vi "GenerateLeftRight.vi"(10 "TrackWidth":dbl=20.0, 11 "SmoothPath":dbl[][](array[numeric])) -> (1 "Right":dbl[][](array[numeric]), 2 "Left":dbl[][](array[numeric]), 3 "Heading":dbl[](array[numeric]))   [LabVIEW 2016]
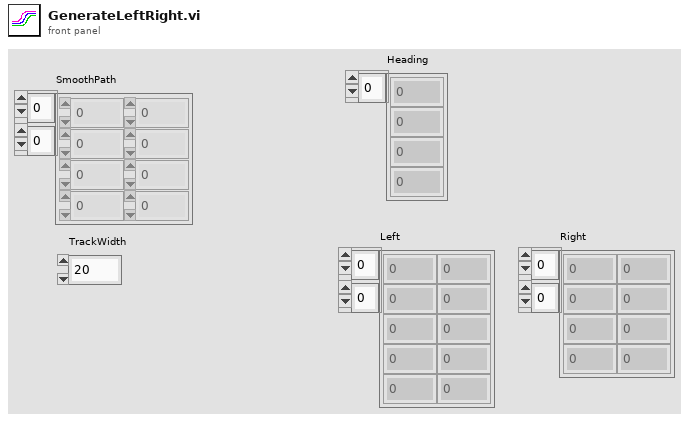
[diagram p1: front panel]
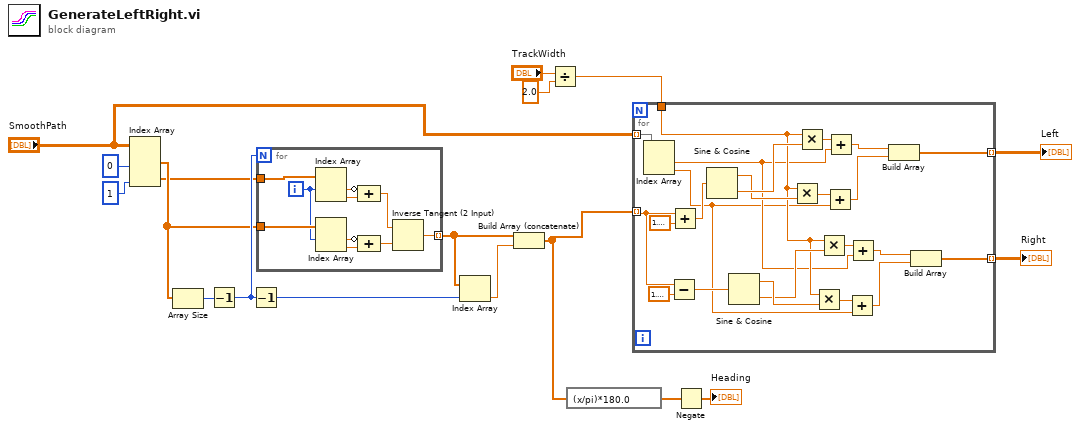
[diagram p0: block diagram]
diagram:
  n1 = Index Array(array="SmoothPath", index (col) #1=0 ("disabled index (col)"), index (col) #2=1 ("index (col)")) -> (element #1=w13:dbl[], element #2=w12:dbl[])  [unwired: 2 in]
  n2 = Array Size(array=w13) -> (size(s)=w17:i32)
  n3 = Decrement(x=w17) -> (x-1=w15:i32)
  n4 = Decrement(x=w15) -> (x-1=w14:i32)
  n5 = for {
    N: w15 -> [_]
    tunnel: w13 -> [w28]
    tunnel: w12 -> [w27]
    tunnel: [w20] -> w5 mode=indexing
    i -> [w19]
    n6 = Index Array(array=w27, index #1=w19) -> (element #1=w25:dbl, element #2=w26:dbl)  [unwired: 1 in]
    n7 = Index Array(array=w28, index #1=w19) -> (element #1=w23:dbl, element #2=w24:dbl)  [unwired: 1 in]
    n8 = Compound Arithmetic op=ADD(invert w25, w26) -> (w22:dbl)
    n9 = Compound Arithmetic op=ADD(invert w23, w24) -> (w21:dbl)
    n10 = Inverse Tangent (2 Input)(1:w21, 2:w22) -> (0:w20:dbl)
  }
  n11 = Index Array(array=w5, index=w14) -> (element=w4:dbl)
  n12 = Build Array (concatenate)(w5, w4) -> (w3:dbl[])
  n13 = Divide(x="TrackWidth", y=2.0) -> (x/y=w9:dbl)
  n14 = expression code="(x/pi)*180.0" ("radians to degrees")(w3) -> (w2:dbl[])
  n15 = for {
    tunnel: w3 -> [w33] mode=indexing
    tunnel: w9 -> [w32]
    tunnel: "SmoothPath" -> [w34] mode=indexing
    tunnel: [w43] -> w7 mode=indexing
    tunnel: [w31] -> w6 mode=indexing
    n16 = Index Array(array=w34) -> (element #1=w30:dbl, element #2=w29:dbl)  [unwired: 2 in]
    n17 = Subtract(x=w33, y=1.5707963267948966) -> (x-y=w36:dbl)
    n18 = Add(x=w33, y=1.5707963267948966) -> (x+y=w50:dbl)
    n19 = Sine & Cosine(0:w50) -> (1:w46:dbl, 2:w47:dbl)
    n20 = Sine & Cosine(0:w36) -> (1:w40:dbl, 2:w39:dbl)
    n21 = Multiply(x=w32, y=w46) -> (x*y=w45:dbl)
    n22 = Multiply(x=w32, y=w47) -> (x*y=w49:dbl)
    n23 = Multiply(x=w32, y=w40) -> (x*y=w41:dbl)
    n24 = Multiply(x=w32, y=w39) -> (x*y=w37:dbl)
    n25 = Add(x=w45, y=w29) -> (x+y=w44:dbl)
    n26 = Add(x=w49, y=w30) -> (x+y=w48:dbl)
    n27 = Add(x=w41, y=w29) -> (x+y=w42:dbl)
    n28 = Add(x=w37, y=w30) -> (x+y=w38:dbl)
    n29 = Build Array(w48, w44) -> (w43:dbl[])
    n30 = Build Array(w38, w42) -> (w31:dbl[])
  }
  "Left" <- w7
  "Right" <- w6
  n31 = Negate(x=w2) -> (-x=→"Heading":dbl[])
